vi "ARC_Comm Get Local Queue Name.vi"(8 "error in":errorcluster caption="错误输入（无错误）", 10 "VI Ref":refnum<vi>) -> (0 "error out":errorcluster caption="错误输出", 1 "VI  Name":string, 2 "VI Ref out":refnum<vi>)   [LabVIEW 2016]
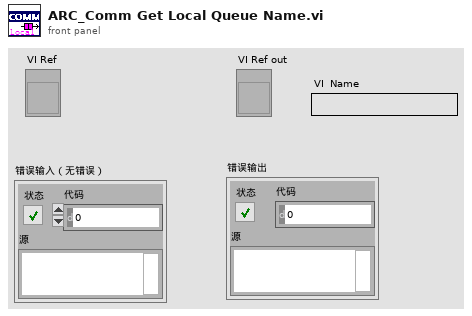
[diagram p1: front panel]
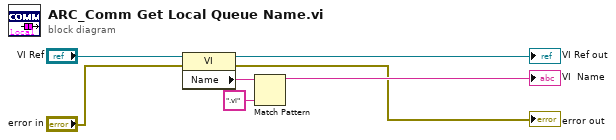
[diagram p0: block diagram]
diagram:
  n1 = property class="VI"(reference="VI Ref", error in="error in") -> (reference out=→"VI Ref out":refnum<vi>, error out=→"error out":errorcluster, "Name"=w5:string)
  n2 = Match Pattern(string=w5, regular expression=".vi" ("正则表达式")) -> (before substring=→"VI  Name":string)  [unwired: 1 in, 3 out]
